vi "Initialize HD44780.vi"(6 "font configuration (5x8 & 2 lines)":T1(ring), 8 "error in (no error)":errorcluster, 9 "number of chips":enum8{"1 chip", "2 chips"}(ring), 10 "device index":i8) -> (0 "error out":errorcluster, 3 "LCD out":u32)   [LabVIEW 2015, in "HD44780 FPGA.lvlib"]
doc: "Initializes character LCD devices that use the Hitachi HD44780 controller. This VI clears the display, sets the cursor to the home position, and sets the entry mode to increment without shift."
uses:
  <vilib>/EmbeddedDisplay/Hitachi HD44780/FPGA/HD44780 FPGA.lvlib
  <vilib>/EmbeddedDisplay/Hitachi HD44780/Common/HD44780 Common.lvlib
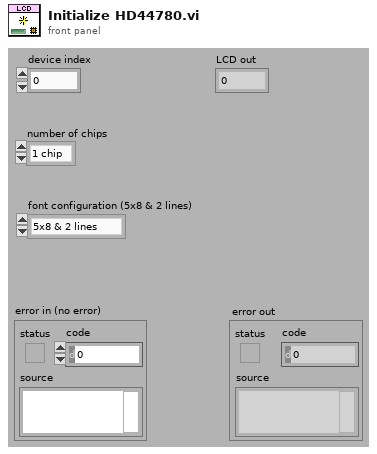
[diagram p1: front panel]
types:
  T1 = enum8{"5x8 & 2 lines", "5x10 & 1 line", "5x8 & 1 line"}
  T2 = enum8{"increment & no shift", "increment & shift", "decrement & no shift", "decrement & shift"}
  T3 = enum8{"cursor off", "cursor on & no blink", "cursor on & blink"}
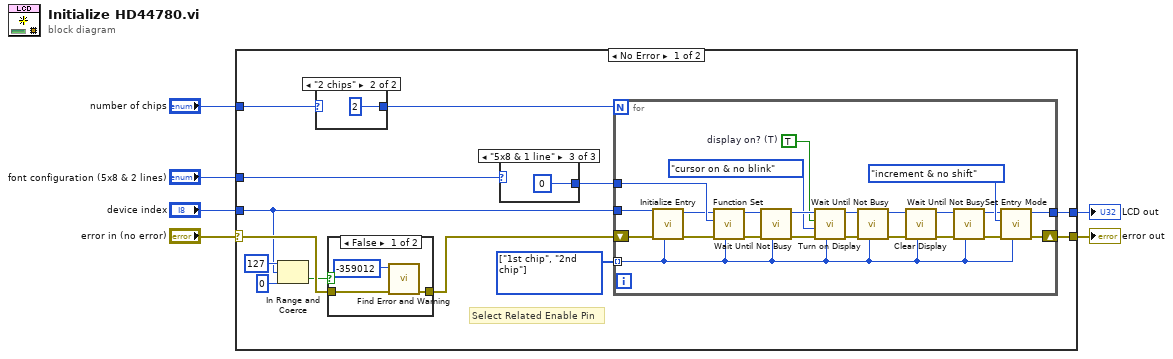
[diagram p0: block diagram]
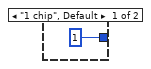
[diagram p2: hidden frame]
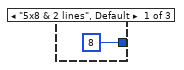
[diagram p4: hidden frame]
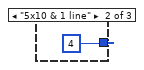
[diagram p5: hidden frame]
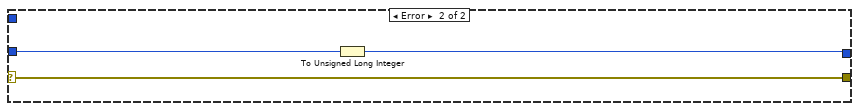
[diagram p6: hidden frame]
diagram:
  n1 = case shown="No Error" "error in (no error)" {
    selector: "error in (no error)" -> [w13 w54]
    tunnel: [w19 w54] -> w6
    tunnel: "device index" -> [w9 w53]
    tunnel: [w18 w52] -> w5
    tunnel: "font configuration (5x8 & 2 lines)" -> [w15 _]
    tunnel: "number of chips" -> [w8 _]
    frame No Error {
      w17 = enum16{"1st chip", "2nd chip"}[] [enum."1st chip", enum."2nd chip"] items=["1st chip", "2nd chip"]
      # "Select Related Enable Pin"
      n2 = In Range and Coerce(upper limit=i8 127, x=w9, lower limit=i8 0) -> (In Range?=w10:bool)  [unwired: 1 out]
      n3 = case shown="\"2 chips\"" w8 {
        tunnel: [1 ("32bit integer") 2 ("32bit integer")] -> w7
        frame "1 chip", Default {
        }
        frame "2 chips" {
        }
      }
      n4 = case shown="False" w10 {
        tunnel: [w23 w25] -> w14
        tunnel: w13 -> [w22 w25]
        frame False {
          n5 = call <vilib>:"Find Error and Warning.vi"("error in (no error)"=w22, "error code"=-359012) -> ("error out"=w23:errorcluster)  [unwired: 9 in]
        }
        frame True {
        }
      }
      n6 = case shown="\"5x8 & 1 line\"" w15 {
        tunnel: [u8 8 u8 4 u8 0] -> w16
        frame "5x8 & 2 lines", Default {
        }
        frame "5x10 & 1 line" {
        }
        frame "5x8 & 1 line" {
        }
      }
      n7 = for {
        N: w7 -> [_]
        tunnel: w17 -> [w31] mode=indexing
        tunnel: w9 -> [w51]
        shift-right: [w35] -> w19
        shift-left: w14 -> [w50]
        tunnel: w16 -> [w49]
        tunnel: [w34] -> w18
        w41 = TRUE  # display on? (T)
        n8 = call <vilib>:"Initialize Entry.vi"("chip select (1st)"=w31, "error in (no error)"=w50, "device index"=w51) -> ("error out"=w48:errorcluster, "LCD out"=w45:u32)  [unwired: 7 in]
        n9 = call <vilib>:"Function Set.vi"("chip select  (1st chip)"=w31, "error in (no error)"=w48, "function set cmd code"=w49, "LCD in"=w45) -> ("error out"=w47:errorcluster, "LCD out"=w46:u32)  [unwired: 6 in]
        n10 = call <vilib>:"Wait Until Not Busy.vi"("chip select  (1st chip)"=w31, "error in (no error)"=w47, "LCD in"=w46) -> ("error out"=w43:errorcluster, "LCD out"=w44:u32)  [unwired: 7 in]
        n11 = call <vilib>:"Turn on Display.vi"("chip select (1st chip)"=w31, "error in (no error)"=w43, "cursor option"=T3."cursor on & no blink" ("cursor option (on & no blink)"), "display on?"=w41, "LCD in"=w44) -> ("error out"=w39:errorcluster, "LCD out"=w40:u32)  [unwired: 5 in]
        n12 = call <vilib>:"Wait Until Not Busy.vi"("chip select  (1st chip)"=w31, "error in (no error)"=w39, "LCD in"=w40) -> ("error out"=w37:errorcluster, "LCD out"=w38:u32)  [unwired: 7 in]
        n13 = call <vilib>:"Clear Display.vi"("chip select (1st chip)"=w31, "error in (no error)"=w37, "LCD in"=w38) -> ("error out"=w32:errorcluster, "LCD out"=w33:u32)  [unwired: 7 in]
        n14 = call <vilib>:"Wait Until Not Busy.vi"("chip select  (1st chip)"=w31, "error in (no error)"=w32, "LCD in"=w33) -> ("error out"=w30:errorcluster, "LCD out"=w29:u32)  [unwired: 7 in]
        n15 = call <vilib>:"Set Entry Mode.vi"("chip select (1st chip)"=w31, "error in (no error)"=w30, "entry mode"=T2."increment & no shift", "LCD in"=w29) -> ("error out"=w35:errorcluster, "LCD out"=w34:u32)  [unwired: 6 in]
      }
    }
    frame Error {
      n16 = To Unsigned Long Integer(number=w53) -> (unsigned 32bit integer=w52:u32)
    }
  }
  "error out" <- w6
  "LCD out" <- w5
